vi "AddUser.vi"(8 "error in (no error)":errorcluster) -> (0 "error out":errorcluster)   [LabVIEW 2021]
uses:
  Controls/UserTypes.ctl
  Controls/UserInfo.ctl
panel:
  in  "User Type":T1 items=["Admin", "Operator"]
  in  "Cancel":bool
  in  "Password":string
  in  "User Name":string
  in  "Add":bool
  in  "Help":bool
  # "Add New User"
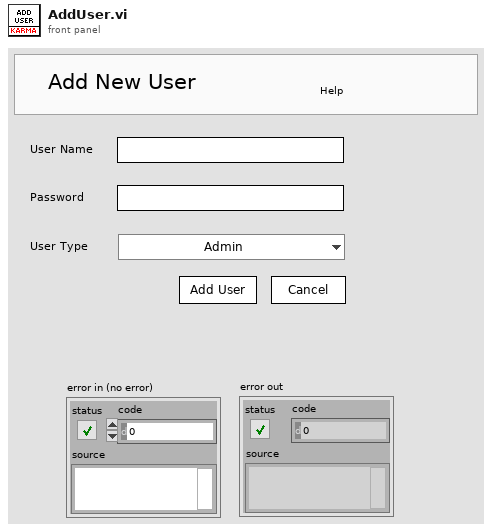
[diagram p1: front panel]
types:
  T1 = typedef "UserTypes.ctl" = u16
  T2 = typedef "UserInfo.ctl" = cluster{"User Name":string, "Password":string, "UserType":T1}
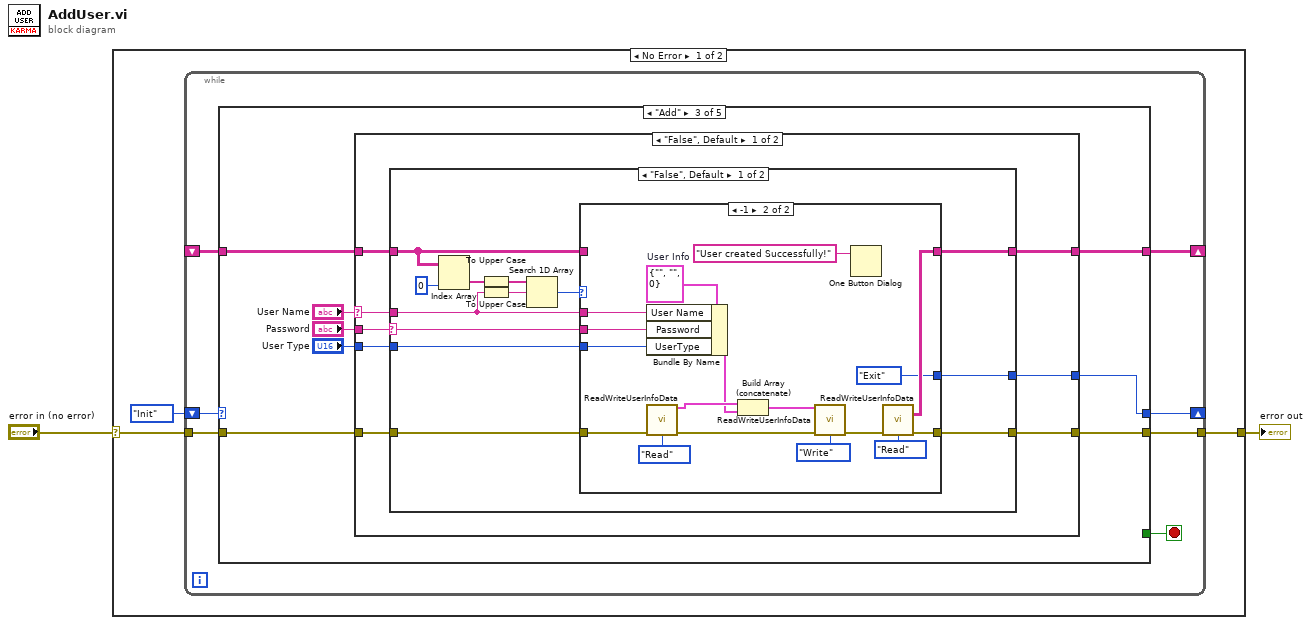
[diagram p0: block diagram]
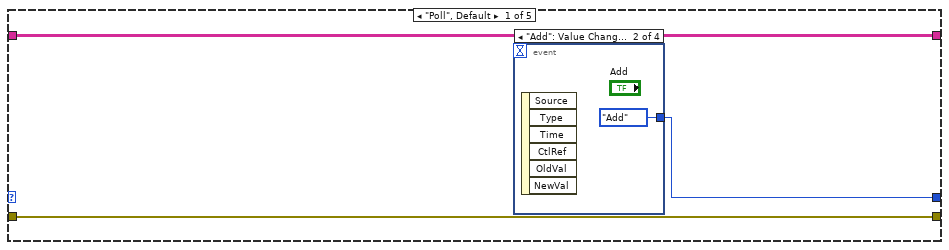
[diagram p2: hidden frame]
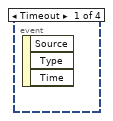
[diagram p3: hidden frame]
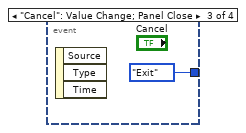
[diagram p4: hidden frame]
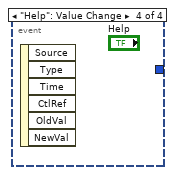
[diagram p5: hidden frame]
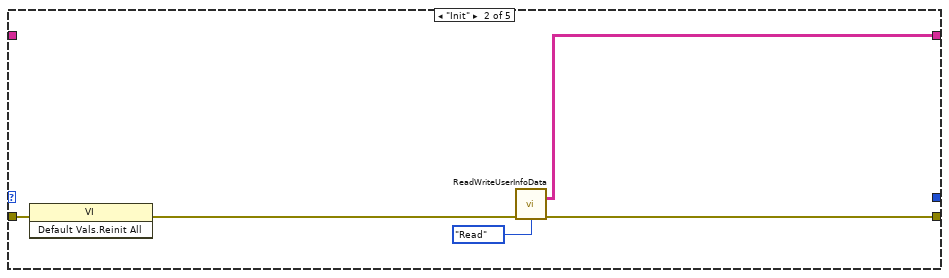
[diagram p6: hidden frame]
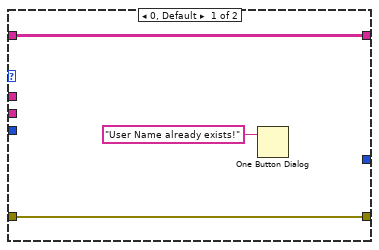
[diagram p7: hidden frame]
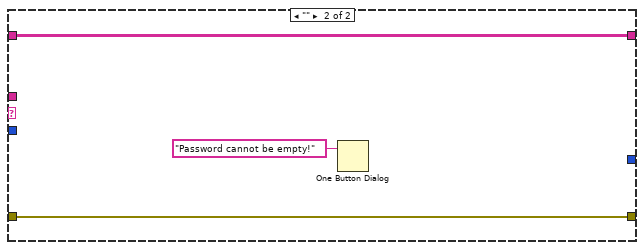
[diagram p8: hidden frame]
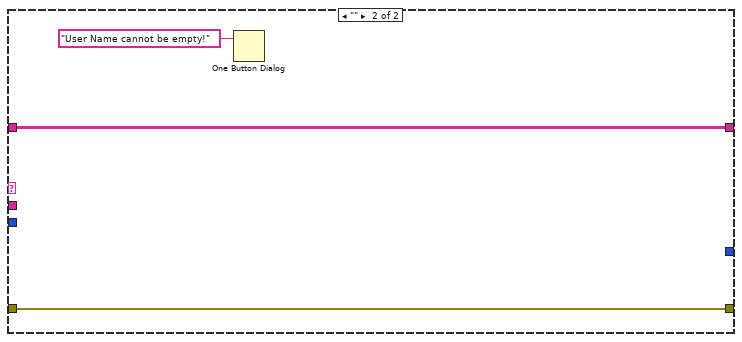
[diagram p9: hidden frame]
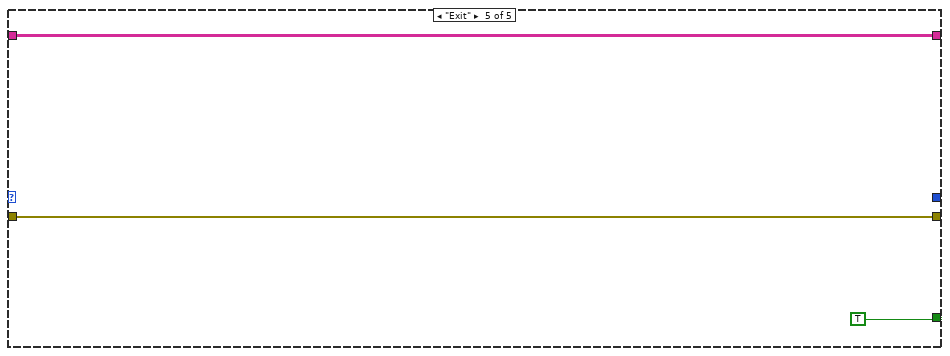
[diagram p11: hidden frame]
diagram:
  n1 = case shown="No Error" "error in (no error)" {
    selector: "error in (no error)" -> [w4 w83]
    tunnel: [w3 w83] -> w1
    frame No Error {
      n2 = while {
        shift-right: [w11] -> _
        shift-left: enum16{"Poll", "Init", "Add", "Error", "Exit"}."Init" -> [w12]
        tunnel: w4 -> [w9]
        tunnel: [w8] -> w3
        shift-right: [w7] -> _
        shift-left: _ -> [w6]
        stop <- w10 stop-if-true
        n3 = case shown="\"Add\"" w12 {
          tunnel: [w15 _ w23 _ _] -> w11
          tunnel: [_ _ _ _ TRUE] -> w10
          tunnel: w9 -> [w13 w22 w26 w79 w81]
          tunnel: [w13 w19 w25 w79 w81] -> w8
          tunnel: [w14 w18 w24 w78 w80] -> w7
          tunnel: w6 -> [w14 _ w28 w78 w80]
          frame "Poll", Default {
            n4 = event shown="[1] \"Add\": Value Change" {
              selector: _ -> [_ _ _ _]
              dyn-events: _ -> [_ _ _ _]
              timeout: _ -> [_ _ _ _]
              tunnel: [_ enum16{"Poll", "Init", "Add", "Error", "Exit"}."Add" enum16{"Poll", "Init", "Add", "Error", "Exit"}."Exit" _] -> w15
              event Timeout {
                n5 = event-data() -> ()  [unwired: 1 in, 3 out]
              }
              event "Add": Value Change {
                n6 = event-data() -> ()  [unwired: 1 in, 6 out]
              }
              event "Cancel": Value Change; Panel Close {
                n7 = event-data() -> ()  [unwired: 1 in, 3 out]
              }
              event "Help": Value Change {
                n8 = event-data() -> ()  [unwired: 1 in, 6 out]
              }
            }
          }
          frame "Init" {
            n9 = invoke class="VI" method="Default Vals.Reinit All"(error in=w22) -> (error out=w21:errorcluster)  [unwired: 2 in, 2 out]
            n10 = call "ReadWriteUserInfoData.vi"("Error in (no error)"=w21, "Operation"=enum16{"Write", "Read"}."Read") -> ("User Info Array out"=w18:string[][], "Error out"=w19:errorcluster)  [unwired: 11 in, 1 out]
          }
          frame "Add" {
            n11 = case shown="\"False\", Default" "User Name" {
              selector: "User Name" -> [w36 _]
              tunnel: "Password" -> [w38 _]
              tunnel: w28 -> [w37 w76]
              tunnel: "User Type" -> [w35 _]
              tunnel: w26 -> [w34 w75]
              tunnel: [w33 w75] -> w25
              tunnel: [w32 w76] -> w24
              tunnel: [w31 _] -> w23
              frame "False", Default {
                n12 = case shown="\"False\", Default" w38 {
                  selector: w38 -> [w45 _]
                  tunnel: w37 -> [w41 w72]
                  tunnel: w36 -> [w46 _]
                  tunnel: w35 -> [w44 _]
                  tunnel: w34 -> [w43 w73]
                  tunnel: [w42 w73] -> w33
                  tunnel: [w40 w72] -> w32
                  tunnel: [w39 _] -> w31
                  frame "False", Default {
                    n13 = Index Array(array=w41, index (col)=0) -> (element=w50:string[])  [unwired: 1 in]
                    n14 = To Upper Case(1:w50) -> (0:w49:string[])
                    n15 = To Upper Case(1:w46) -> (0:w48:string)
                    n16 = Search 1D Array(1D array=w49, element=w48) -> (index of element=w47:i32)  [unwired: 1 in]
                    n17 = case shown="-1" w47 {
                      tunnel: w46 -> [_ w70]
                      tunnel: w45 -> [_ w69]
                      tunnel: w44 -> [_ w68]
                      tunnel: w43 -> [w53 w63]
                      tunnel: [w53 w58] -> w42
                      tunnel: w41 -> [w52 _]
                      tunnel: [w52 w56] -> w40
                      tunnel: [_ enum16{"Poll", "Init", "Add", "Error", "Exit"}."Exit"] -> w39
                      frame 0, Default {
                        n18 = One Button Dialog(message="User Name already exists!") -> ()  [unwired: 1 in, 1 out]
                      }
                      frame -1 {
                        w71 = T2 {"User Name"="", "Password"="", "UserType"=0}  # User Info
                        n19 = Bundle By Name(cluster=w71, "User Name"=w70, "Password"=w69, "UserType"=w68) -> (w66:T2)
                        n20 = call "ReadWriteUserInfoData.vi"("Error in (no error)"=w63, "Operation"=enum16{"Write", "Read"}."Read") -> ("User Info Array of Clusters Out"=w67:T2[], "Error out"=w62:errorcluster)  [unwired: 11 in, 1 out]
                        n21 = Build Array (concatenate)(w67, w66) -> (w65:T2[])
                        n22 = call "ReadWriteUserInfoData.vi"("User Info  Array In"=w65, "Error in (no error)"=w62, "Operation"=enum16{"Write", "Read"}."Write") -> ("Error out"=w59:errorcluster)  [unwired: 10 in, 2 out]
                        n23 = One Button Dialog(message="User created Successfully!") -> ()  [unwired: 1 in, 1 out]
                        n24 = call "ReadWriteUserInfoData.vi"("Error in (no error)"=w59, "Operation"=enum16{"Write", "Read"}."Read") -> ("User Info Array out"=w56:string[][], "Error out"=w58:errorcluster)  [unwired: 11 in, 1 out]
                      }
                    }
                  }
                  frame "" {
                    n25 = One Button Dialog(message="Password cannot be empty!") -> ()  [unwired: 1 in, 1 out]
                  }
                }
              }
              frame "" {
                n26 = One Button Dialog(message="User Name cannot be empty!") -> ()  [unwired: 1 in, 1 out]
              }
            }
          }
          frame "Error" {
          }
          frame "Exit" {
          }
        }
      }
    }
    frame Error {
    }
  }
  "error out" <- w1
